vi "myRIOXC Picture Resize.vi"(8 "image data":T1, 10 "XCtrl Reference":refnum<vi>, 11 "picture":picture) -> (3 "new picture":picture)   [LabVIEW 2021]
uses:
  <vilib>/picture/picture.llb/imagedata.ctl
  <vilib>/picture/picture.llb/Draw True-Color Pixmap.vi
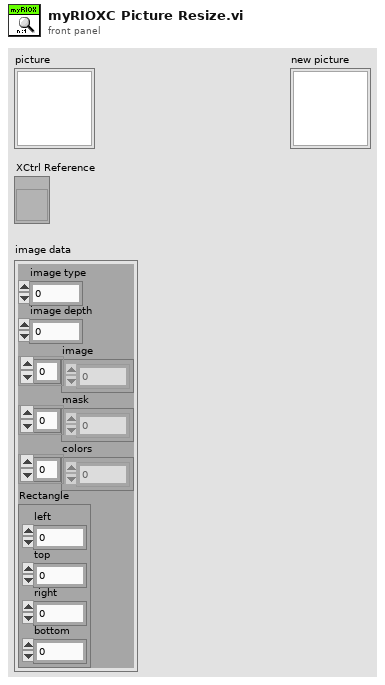
[diagram p1: front panel]
types:
  T1 = typedef "imagedata.ctl" = cluster{"image type":i32, "image depth":i32, "image":u8[], "mask":u8[], "colors":u32[], "Rectangle":cluster{"left":i16, "top":i16, "right":i16, "bottom":i16}}
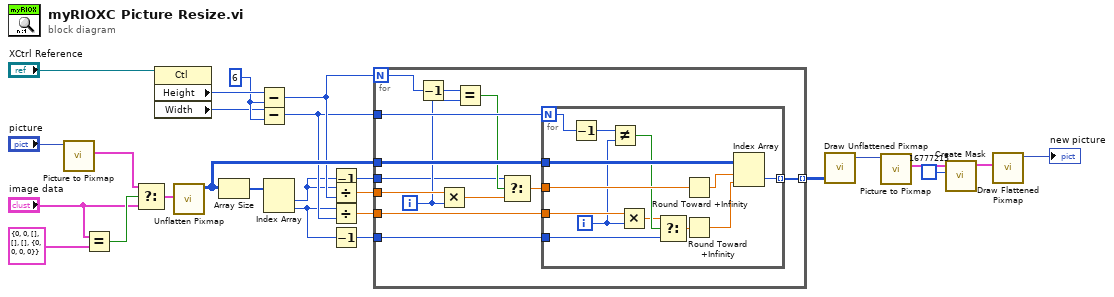
[diagram p0: block diagram]
diagram:
  w12 = u32 6 ("y")
  n1 = call <vilib>:"Picture to Pixmap.vi"("picture"="picture") -> ("image data"=w20:T1)  [unwired: 9 in, 1 out]
  n2 = Equal?(x="image data", y=T1 {"image type"=0, "image depth"=0, "image"=[], "mask"=[], "colors"=[], "Rectangle"={"left"=0, "top"=0, "right"=0, "bottom"=0}} ("image data")) -> (x = y?=w21:bool)
  n3 = Select(t=w20, s=w21, f="image data") -> (s? t:f=w18:T1)
  n4 = property class="Ctl"(reference="XCtrl Reference") -> ("Height"=w13:u32, "Width"=w11:u32)  [unwired: 1 in, 2 out]
  n5 = call <vilib>:"Unflatten Pixmap.vi"("image data"=w18) -> ("24-bit pixmap"=w26:u32[][])  [unwired: 4 in, 6 out]
  n6 = Array Size(array=w26) -> (size(s)=w25:i32[])
  n7 = Subtract(x=w13, y=w12) -> (x-y=w10:u32)
  n8 = Subtract(x=w11, y=w12) -> (x-y=w9:u32)
  n9 = Index Array(array=w25) -> (element #1=w8:i32, element #2=w7:i32)  [unwired: 2 in]
  n10 = Decrement(x=w8) -> (x-1=w6:i32)
  n11 = Divide(x=w8, y=w10) -> (x/y=w24:dbl)
  n12 = Divide(x=w7, y=w9) -> (x/y=w23:dbl)
  n13 = Decrement(x=w7) -> (x-1=w5:i32)
  n14 = for {
    N: w10 -> [w34]
    tunnel: w26 -> [w39]
    tunnel: [w38] -> w22 mode=indexing
    tunnel: w9 -> [w35]
    tunnel: w24 -> [w37]
    tunnel: w23 -> [w36]
    tunnel: w6 -> [w30]
    tunnel: w5 -> [w27]
    i -> [w31]
    n15 = Decrement(x=w34) -> (x-1=w32:i32)
    n16 = Multiply(x=w37, y=w31) -> (x*y=w28:dbl)
    n17 = Equal?(x=w32, y=w31) -> (x = y?=w33:bool)
    n18 = Select(t=w30, s=w33, f=w28) -> (s? t:f=w29:dbl)
    n19 = for {
      N: w35 -> [w46]
      tunnel: w39 -> [w52]
      tunnel: [w51] -> w38 mode=indexing
      tunnel: w29 -> [w48]
      tunnel: w36 -> [w50]
      tunnel: w27 -> [w42]
      i -> [w44]
      n20 = Decrement(x=w46) -> (x-1=w45:i32)
      n21 = Not Equal?(x=w45, y=w44) -> (x != y?=w43:bool)
      n22 = Multiply(x=w50, y=w44) -> (x*y=w41:dbl)
      n23 = Select(t=w41, s=w43, f=w42) -> (s? t:f=w40:dbl)
      n24 = Round Toward +Infinity(x=w48) -> (ceil(x): smallest int >= x=w47:dbl)
      n25 = Round Toward +Infinity(x=w40) -> (ceil(x): smallest int >= x=w49:dbl)
      n26 = Index Array(array=w52, index (row)=w47, index (col)=w49) -> (element=w51:u32)
    }
  }
  n27 = call-poly <vilib>:"Draw Unflattened Pixmap.vi"("data (RGB format)"=w22) -> ("new picture"=w16:picture)  [unwired: 8 in]
  n28 = call <vilib>:"Picture to Pixmap.vi"("picture"=w16) -> ("image data"=w15:T1)  [unwired: 9 in, 1 out]
  n29 = call <vilib>:"Create Mask.vi"("Mask Color (Black)"=u32 16777215, "image data"=w15) -> ("image data"=w17:T1)  [unwired: 9 in]
  n30 = call <vilib>:"Draw Flattened Pixmap.vi"("image data"=w17) -> ("new picture"=→"new picture":picture)  [unwired: 8 in]
